vi "Execute Command.vi"(8 "error in (no error)":errorcluster, 10 "command":T1={"Command"=enum."Rx", "Parameters"={"arg1"=0, "arg2"=0}}, 11 "Dispatcher in":refnum<class "Dispatcher Thread.lvclass">) -> (0 "error out":errorcluster, 3 "Dispatcher out":refnum<class "Dispatcher Thread.lvclass">)   [LabVIEW 2017, in "DSF Core.lvlib" / "Dispatcher Thread.lvclass"]
uses:
  Dispatcher Thread.lvclass
  Interfaces/Dispatcher/Command Data.ctl
  Interfaces/Dispatcher/Command.ctl
  Interfaces/Dispatcher/Parameters.ctl
  Interfaces/Dispatcher/Dispatcher Interface.lvclass
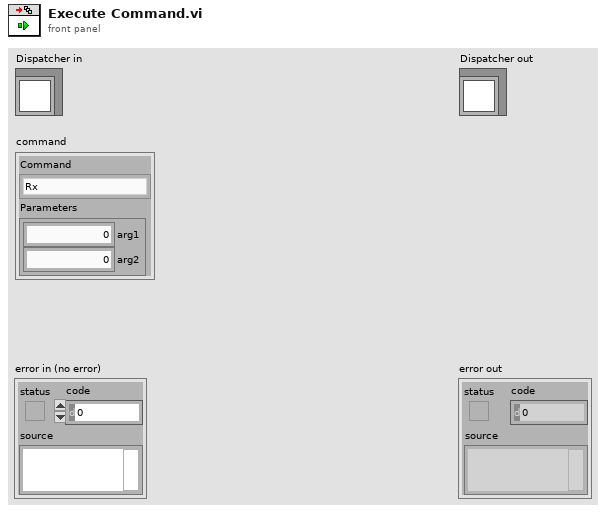
[diagram p1: front panel]
types:
  T1 = typedef "DSF Core.lvlib/Dispatcher Interface.lvclass/Command Data.ctl" = cluster{"Command":T2, "Parameters":T3}
  T2 = typedef "DSF Core.lvlib/Dispatcher Interface.lvclass/Command.ctl" = enum8{"Start", "Rx", "Tx", "Set Inline Buffer", "Shutdown"}
  T3 = typedef "DSF Core.lvlib/Dispatcher Interface.lvclass/Parameters.ctl" = cluster{"arg1":u64, "arg2":u64}
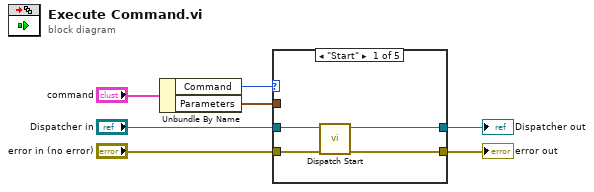
[diagram p0: block diagram]
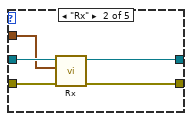
[diagram p2: hidden frame]
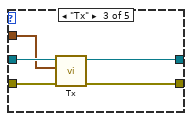
[diagram p3: hidden frame]
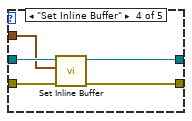
[diagram p4: hidden frame]
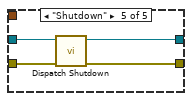
[diagram p5: hidden frame]
diagram:
  n1 = Unbundle By Name("command") -> ("Command"=w2:T2, "Parameters"=w1:T3)
  n2 = case shown="\"Start\"" w2 {
    tunnel: "Dispatcher in" -> [w11 w16 w21 w25 w30]
    tunnel: [w9 w14 w19 w23 w28] -> w6
    tunnel: "error in (no error)" -> [w10 w15 w20 w26 w29]
    tunnel: [w8 w13 w18 w22 w27] -> w5
    tunnel: w1 -> [_ w12 w17 w24 _]
    frame "Start" {
      n3 = call "Dispatch Start.vi"("error in (no error)"=w10, "Dispatcher in"=w11) -> ("error out"=w8:errorcluster, "Dispatcher out"=w9:refnum<class "Dispatcher Thread.lvclass">)  [unwired: 8 in]
    }
    frame "Rx" {
      n4 = call "Rx.vi"("error in (no error)"=w15, "Command Parameters"=w12, "Dispatcher in"=w16) -> ("error out"=w13:errorcluster, "Dispatcher out"=w14:refnum<class "Dispatcher Thread.lvclass">)  [unwired: 7 in]
    }
    frame "Tx" {
      n5 = call "Tx.vi"("error in (no error)"=w20, "Command Parameters"=w17, "Dispatcher in"=w21) -> ("error out"=w18:errorcluster, "Dispatcher out"=w19:refnum<class "Dispatcher Thread.lvclass">)  [unwired: 7 in]
    }
    frame "Set Inline Buffer" {
      n6 = call "Set Inline Buffer.vi"("error in (no error)"=w26, "Command Parameters"=w24, "Dispatcher in"=w25) -> ("error out"=w22:errorcluster, "Dispatcher out"=w23:refnum<class "Dispatcher Thread.lvclass">)  [unwired: 7 in]
    }
    frame "Shutdown" {
      n7 = call "Dispatch Shutdown.vi"("error in (no error)"=w29, "Dispatcher in"=w30) -> ("error out"=w27:errorcluster, "Dispatcher out"=w28:refnum<class "Dispatcher Thread.lvclass">)  [unwired: 8 in]
    }
  }
  "error out" <- w5
  "Dispatcher out" <- w6
